vi "PH_PILS.Action _Submode.vi"(0 "i ref in":refnum<vi>, 5 "error IO":errorcluster) -> (14 "i ref out":refnum<vi>, 19 "error out":errorcluster)   [LabVIEW 2014, in "PH_PILS.lvlib"]
doc: "This Vi calculates the submode."
uses:
  PH_PILS.lvlib
  PH_PILS.Operation Mode.ctl
  PH_Basics/PH_Common/PH_Common.lvlib
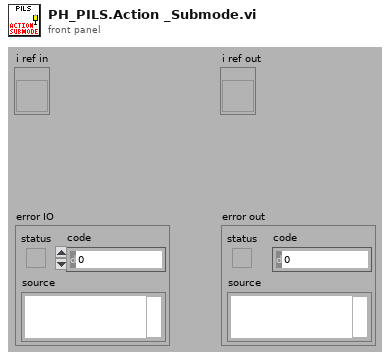
[diagram p1: front panel]
types:
  T1 = typedef "PH_PILS.lvlib/PH_PILS.i attribute.ctl" = cluster{"Boolean":cluster{"GUI Ref":refnum<vi>, "Status":i32}[], "GUI Refs Exp. Shutters":cluster{"1":refnum<vi>, "2":refnum<vi>, "3":refnum<vi>, "4":refnum<vi>}, "Tristate2Run GUI Refs":refnum<vi>[], "EO-Likes":cluster{"GUI Ref":refnum<vi>, "Status":i32}[], "Operation Mode":cluster{"Operation Mode":T2, "GUI":cluster{"Ref State":refnum<vi>, "Ref":refnum<vi>}, "Servicemode":cluster{"Tagname":string, "Status":i32}, "Labormode":cluster{"Tagname":string, "Status":i32}, "Searchmode":cluster{"Tagname":string, "Status":i32}, "Shotmode":cluster{"Tagname":string, "Status":i32}}, "Submode":cluster{"Submode":T3, "GUI":cluster{"Ref State":refnum<vi>, "Ref":refnum<vi>}, "Submode":cluster{"Tagname":string, "Status":i32}}, "Experiment":cluster{"Experiment":enum16{"unknown", "intern", "4 (Z6)", "3", "2", "1"}, "GUI":cluster{"Ref State":refnum<vi>, "Ref":refnum<vi>}, "intern":cluster{"Tagname":string, "Status":i32}, "Exp 4":cluster{"Tagname":string, "Status":i32}, "Exp 3":cluster{"Tagname":string, "Status":i32}, "Exp 2":cluster{"Tagname":string, "Status":i32}, "Exp 1":cluster{"Tagname":string, "Status":i32}}, "TristateNormal":cluster{"GUI Ref":refnum<vi>, "Status":i32}[], "Door Tags":cluster{"GUI Ref":refnum<vi>, "Status":i32}[], "GUIlessTags":cluster{"Name":string, "Status":i32}[], "Beamline GUI Refs":refnum<vi>[], "Special Boolean":cluster{"GUI Ref":refnum<vi>, "Status":i32}[], "Laserpower":cluster{"GUI Ref":refnum<vi>, "Status":i32}[], "Shutter":cluster{"GUI Ref":refnum<vi>, "Status":i32}[], "Tristate EO Like":cluster{"GUI Ref":refnum<vi>, "Status":i32}[], "PP":cluster{"GUI Ref":refnum<vi>, "Status":i32, "Head Ref":refnum<vi>, "Slider Ref":refnum<vi>}[], "Switch Knobs":cluster{"GUI Ref":refnum<vi>, "Status":i32}[], "Latch Knob GUI Refs":refnum<vi>[], "FailureCounter":i32, "Enabled Status":cluster{"Laser":i32, "PreAmp":i32, "MainAmp":i32}, "Mercury":refnum<vi>, "Instance Rods":string, "Logfile":path, "Beckhoff-Instance Internal":string, "Beckhoff-Instance External":string, "Enabling Rights":cluster{"Name":string, "Password":string, "PA?":bool, "MA?":bool, "Exp?":bool}[]}
  T2 = typedef "PH_PILS.lvlib/PH_PILS.Operation Mode.ctl" = enum16{"unknown", "Service", "Labor", "Search", "Shot"}
  T3 = typedef "PH_PILS.lvlib/PH_PILS.Submode.ctl" = enum16{"unknown", "HV-Normal", "HV-Test"}
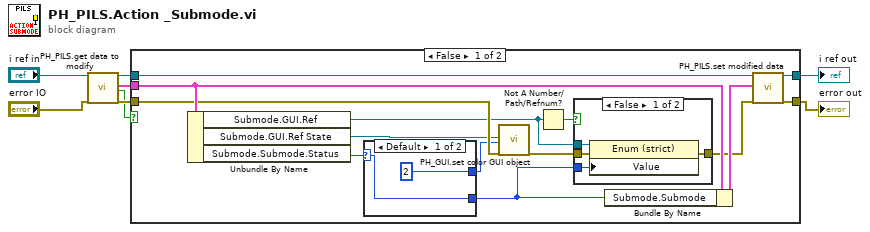
[diagram p0: block diagram]
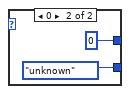
[diagram p2: hidden frame]
diagram:
  n1 = call "PH_PILS.get data to modify.vi"("i ref in"="i ref in", "error in (no error)"="error IO") -> ("i ref out"=w7:refnum<vi>, "i attribute"=w5:T1, "timed out"=w6:bool, "error out"=w8:errorcluster)  [unwired: 14 in]
  n2 = case shown="False" w6 {
    tunnel: [w22 w32] -> w3
    tunnel: w8 -> [w17 w32]
    tunnel: [w21 w33] -> w4
    tunnel: w7 -> [w20 w33]
    tunnel: w5 -> [w19 _]
    frame False {
      n3 = Unbundle By Name(w19) -> ("Submode.GUI.Ref"=w12:refnum<vi>, "Submode.GUI.Ref State"=w13:refnum<vi>, "Submode.Submode.Status"=w9:i32)
      n4 = case shown="Default" w9 {
        selector: w9 -> [w23 _]
        tunnel: [w23 PH_PILS.Operation_Mode."unknown" ("Operation Mode.Operation Mode")] -> w11
        tunnel: [2 ("State") 0 ("State")] -> w10
        frame Default {
        }
        frame 0 {
        }
      }
      n5 = call "PH_GUI.set color GUI object.vi"("GUI object Ref"=w13, "State"=w10, "error in (no error)"=w17) -> ("error out"=w14:errorcluster)  [unwired: 16 in]
      n6 = Not A Number/Path/Refnum?(number/path/refnum=w12) -> (NaN/Path/Refnum?=w15:bool)
      n7 = case shown="False" w15 {
        tunnel: w14 -> [w30 w31]
        tunnel: [w29 w31] -> w16
        tunnel: w12 -> [w28 _]
        tunnel: w11 -> [w27 _]
        frame False {
          n8 = property class="Enum (strict)"(reference=w28, error in=w30, "Value"=w27) -> (error out=w29:errorcluster)  [unwired: 1 out]
        }
        frame True {
        }
      }
      n9 = Bundle By Name(cluster=w19, "Submode.Submode"=w11) -> (w18:T1)
      n10 = call "PH_PILS.set modified data.vi"("i ref in"=w20, "i attribute"=w18, "error in (no error)"=w16) -> ("i ref out"=w21:refnum<vi>, "error out"=w22:errorcluster)  [unwired: 15 in]
    }
    frame True {
    }
  }
  "error out" <- w3
  "i ref out" <- w4
